vi "SE_HV200.ErrorBypass.vi"(7 "error in (no error)":errorcluster) -> (8 "error out":errorcluster)   [LabVIEW 2014, in "SE_HV200.lvlib"]
uses:
  SE_HV200.lvlib
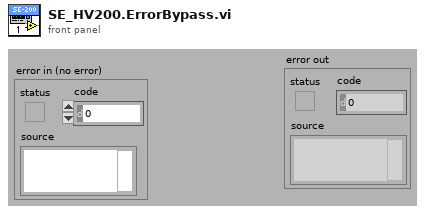
[diagram p1: front panel]
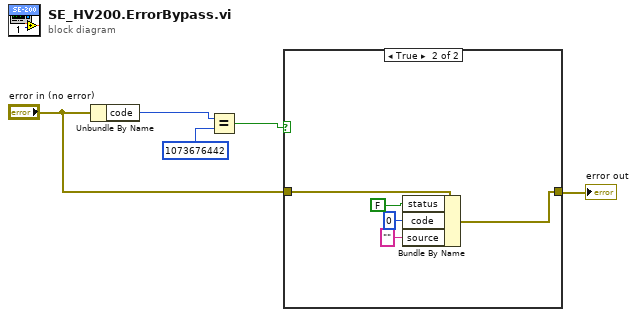
[diagram p0: block diagram]
diagram:
  n1 = Unbundle By Name("error in (no error)") -> ("code"=w4:i32)
  n2 = Equal?(x=w4, y=1073676442) -> (x = y?=w3:bool)
  n3 = case shown="True" w3 {
    tunnel: "error in (no error)" -> [w6 w11]
    tunnel: [w6 w10] -> w1
    frame False {
    }
    frame True {
      n4 = Bundle By Name(cluster=w11, "status"=FALSE, "code"=0, "source"="") -> (w10:errorcluster)
    }
  }
  "error out" <- w1
